vi "Delete Instrument Addon.vi"(8 "error in (no error)":errorcluster, 11 "instrument addon refnum":T1=18446744073709551615 format="%.0x") -> (0 "error out":errorcluster)   [LabVIEW 2018, in "Instrument Addon Scripting API.lvlib"]
doc: "Deletes the specified Instrument Addon Custom Device."
uses:
  Instrument Addon Scripting API.lvlib
  <vilib>/NI Veristand/Custom Device API/Custom Device Item Ref.ctl
  <vilib>/NI Veristand/Custom Device API/Custom Device API.lvlib
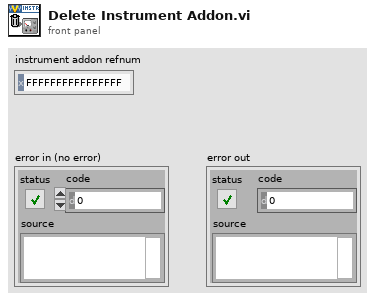
[diagram p1: front panel]
types:
  T1 = typedef "Custom Device API.lvlib/Custom Device Item Ref.ctl" = u64
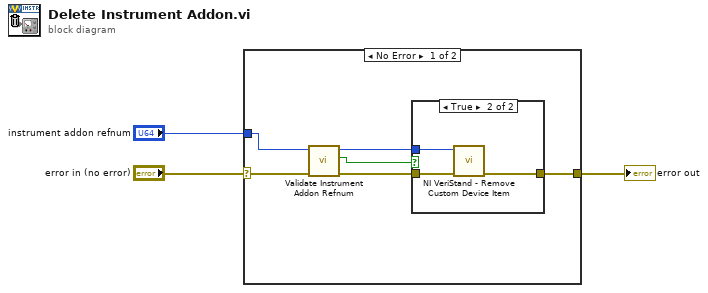
[diagram p0: block diagram]
diagram:
  n1 = case shown="No Error" "error in (no error)" {
    selector: "error in (no error)" -> [w8 w14]
    tunnel: "instrument addon refnum" -> [w4 _]
    tunnel: [w9 w14] -> w3
    frame No Error {
      n2 = call "Validate Instrument Addon Refnum.vi"("Error In"=w8, "Refnum In"=w4) -> ("Error Out"=w5:errorcluster, "Is Instrument Addon?"=w7:bool, "Refnum Out"=w6:T1)  [unwired: 7 in]
      n3 = case shown="True" w7 {
        tunnel: [w10 w13] -> w9
        tunnel: w6 -> [_ w12]
        tunnel: w5 -> [w10 w11]
        frame False {
        }
        frame True {
          n4 = call <vilib>:"NI VeriStand - Remove Custom Device Item.vi"("error in (no error)"=w11, "Item Ref in"=w12) -> ("error out"=w13:errorcluster)  [unwired: 8 in, 1 out]
        }
      }
    }
    frame Error {
    }
  }
  "error out" <- w3
